vi "Read Time Entry.vi"(8 "error in (no error)":errorcluster, 10 "GUID":string, 11 "Time Entries in":refnum<class "Time Entries.lvclass">) -> (0 "error out":errorcluster, 3 "Time Entries out":refnum<class "Time Entries.lvclass">)   [LabVIEW 2020, in "Time Entries.lvclass"]
doc: "VI for override that will read the specific time entry from the file/database/other specified for record keeping. The GUID is used because that is a unique way of identifying an entry.\n\n04/2025 Erich Schlieper"
uses:
  Time Entries.lvclass
  Time Entries.lvclass/Time Entries.ctl
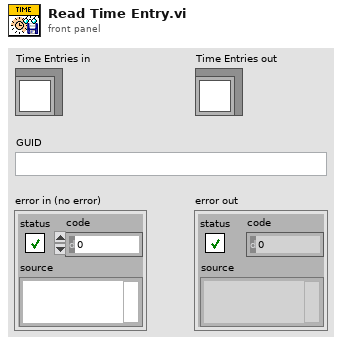
[diagram p1: front panel]
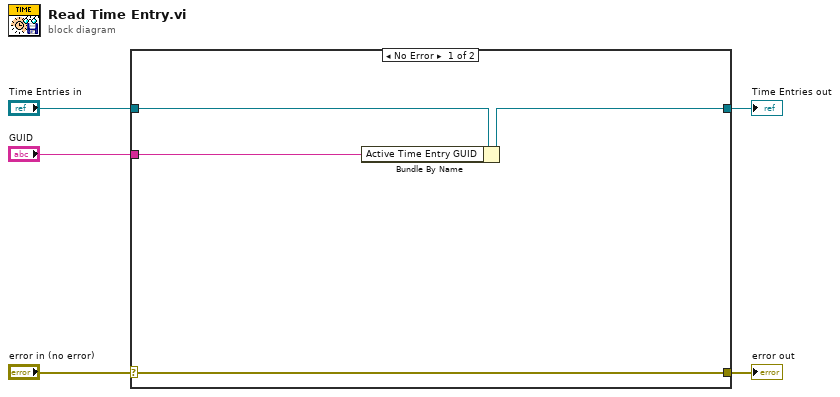
[diagram p0: block diagram]
diagram:
  n1 = case shown="No Error" "error in (no error)" {
    selector: "error in (no error)" -> [w8 w11]
    tunnel: [w8 w11] -> w4
    tunnel: [w7 w10] -> w2
    tunnel: "Time Entries in" -> [w9 w10]
    tunnel: "GUID" -> [w6 _]
    frame No Error {
      n2 = Bundle By Name(cluster=w9, "Active Time Entry GUID"=w6) -> (w7:refnum<class "Time Entries.lvclass">)
    }
    frame Error {
    }
  }
  "error out" <- w4
  "Time Entries out" <- w2
